vi "Fetch Waveform.vi"(8 "error in (no error)":errorcluster, 9 "Timeout(ms)":i32=5000 caption="Maximum Time (5000)", 10 "Number of Channels":i32, 11 "VISA resource name":refnum<visa-resource-name>) -> (0 "error out":errorcluster, 1 "wfm info GEECS":T1(array[cluster]), 2 "I16 Out":i16[][](array[numeric]), 3 "VISA resource name out":refnum<visa-resource-name>, 5 "Scaled Waveform":waveform(dbl)[](array[waveform]))   [LabVIEW 2020]
uses:
  Rohde&Schwarz RTx Oscilloscopes.lvlib
panel:
  out "Output array":i16[](array[numeric])
  out "Waveform":waveform(dbl)
  out "waveform info":T2
  out "Actual Points":i32
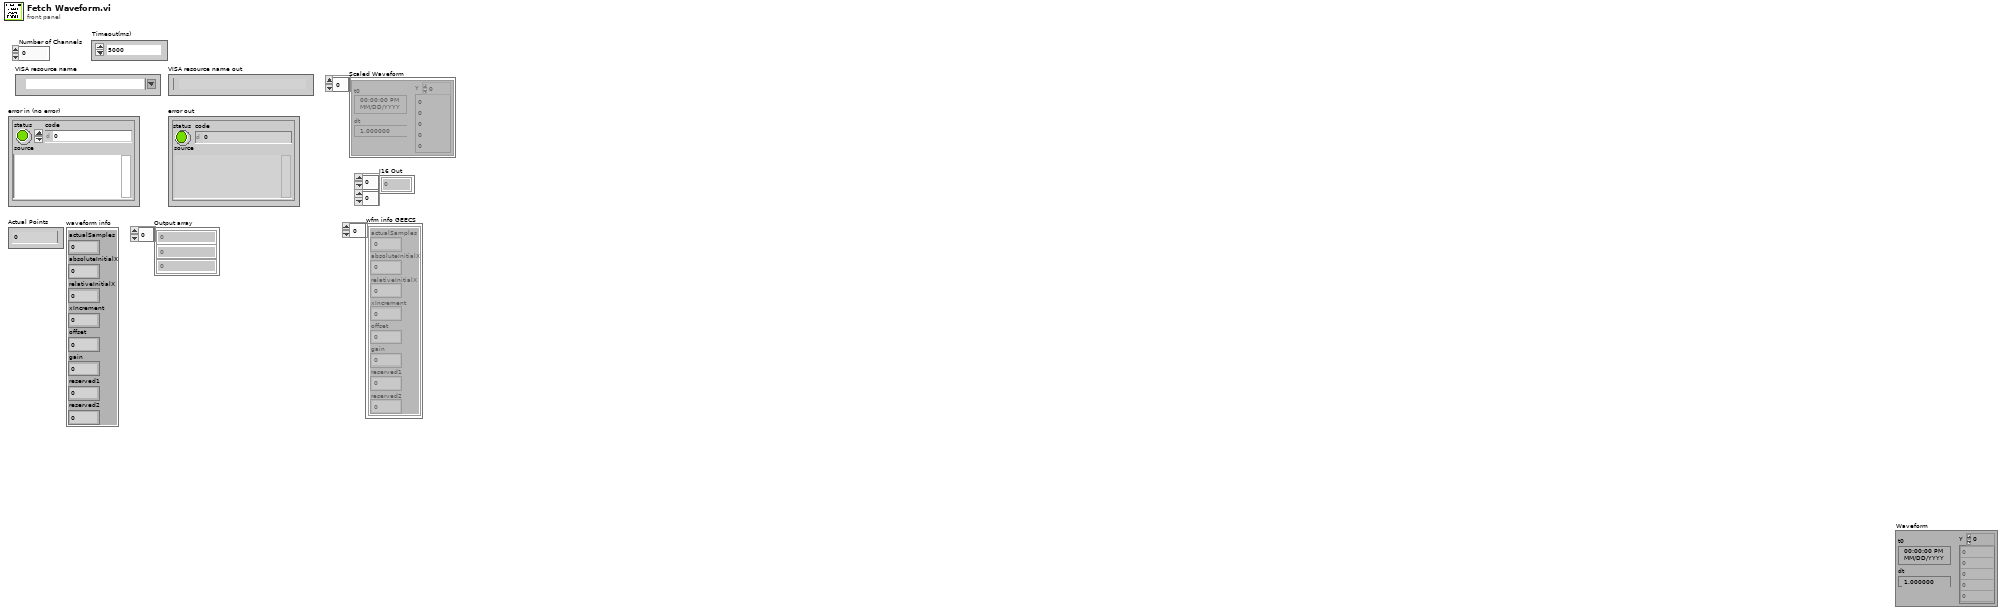
[diagram p1: front panel]
types:
  T1 = cluster{"actualSamples":i32, "absoluteInitialX":dbl, "relativeInitialX":dbl, "xIncrement":dbl, "offset":dbl, "gain":dbl, "reserved1":dbl, "reserved2":dbl}[]
  T2 = cluster{"actualSamples":i32, "absoluteInitialX":dbl, "relativeInitialX":dbl, "xIncrement":dbl, "offset":dbl, "gain":dbl, "reserved1":dbl, "reserved2":dbl}
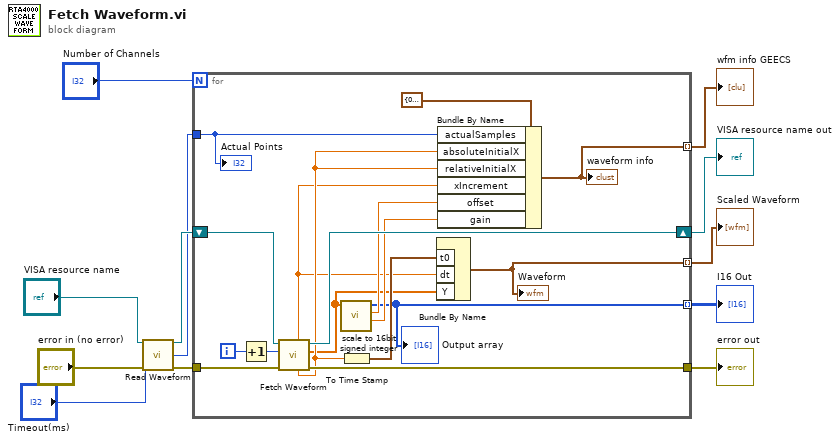
[diagram p0: block diagram]
diagram:
  n1 = call "Read Waveform.vi"("VISA resource name"="VISA resource name", "Maximum Time (5000)"="Timeout(ms)", "error in (no error)"="error in (no error)") -> ("VISA resource name out"=w12:refnum<visa-resource-name>, "Actual Points"=w5:i32, "error out"=w6:errorcluster)  [unwired: 7 in, 3 out]
  n2 = for {
    N: "Number of Channels" -> [_]
    tunnel: [w28] -> w9
    shift-right: [w27] -> w8
    shift-left: w12 -> [w29]
    tunnel: w6 -> [w26]
    tunnel: w5 -> [w22]
    tunnel: [w15] -> w4 mode=indexing
    tunnel: [w14] -> w3 mode=indexing
    tunnel: [w13] -> w2 mode=indexing
    i -> [w25]
    n3 = Increment(x=w25) -> (x+1=w24:i32)
    n4 = call "Fetch Waveform.vi"("error in (no error)"=w26, "Channel (1)"=w24, "VISA resource name"=w29) -> ("error out"=w28:errorcluster, "Waveform Array"=w16:dbl[], "VISA resource name out"=w27:refnum<visa-resource-name>, "Initial X"=w18:dbl, "X Increment"=w17:dbl)  [unwired: 4 in]
    n5 = call "scale to 16bit signed integer.vi"("Waveform Array"=w16) -> ("gain"=w20:dbl, "offset"=w21:dbl, "Output array"=w13:i16[])  [unwired: 8 in]
    "Output array" <- w13
    n6 = To Time Stamp(1:w18) -> (0:w19:timestamp)
    n7 = Bundle By Name("t0"=w19, "dt"=w17, "Y"=w16) -> (w15:waveform(dbl))  [unwired: 1 in]
    "Waveform" <- w15
    n8 = Bundle By Name(cluster=T2 {"actualSamples"=0, "absoluteInitialX"=0.0, "relativeInitialX"=0.0, "xIncrement"=0.0, "offset"=0.0, "gain"=0.0, "reserved1"=0.0, "reserved2"=0.0} ("element"), "actualSamples"=w22, "absoluteInitialX"=w18, "relativeInitialX"=w18, "xIncrement"=w17, "offset"=w21, "gain"=w20) -> (w14:T2)
    "waveform info" <- w14
    "Actual Points" <- w22
  }
  "error out" <- w9
  "VISA resource name out" <- w8
  "Scaled Waveform" <- w4
  "wfm info GEECS" <- w3
  "I16 Out" <- w2
